vi "Dark Current Test Remastered Test Run.vi"() -> ()   [LabVIEW 2020]
uses:
  <instrlib>/CAEN PSM/CAEN PSM.lvlib
  <vilib>/Utility/file.llb/Write Delimited Spreadsheet (string).vi
  <vilib>/Utility/file.llb/Write Delimited Spreadsheet (DBL).vi
panel:
  out "7 4":bool
  out "6 4":bool
  out "8 4":bool
  out "5 4":bool
  out "4 4":bool
  out "3 4":bool
  out "2 4":bool
  out "1 4":bool
  out "Test is Running 4":bool
  out "OVV? 8":bool=TRUE
  out "OVC? 8":bool=TRUE
  out "Actual Voltage Level (V) 8":dbl format="%#_13g"
  out "Actual Current Limit (nA) 4":dbl format="%#_13g"
  in  "dt (s) 4":i32
  out "Time Left (s) 4":dbl
  out "Power Supply Trip 4":bool
  in  "N 4":i32
  in  "Channel # 4":i32
  in  "VISA resource name 4":refnum<visa-resource-name>
  out "OVV? 7":bool=TRUE
  out "OVC? 7":bool=TRUE
  out "Actual Voltage Level (V) 7":dbl format="%#_13g"
  out "Recorded Current\nfor Previous Tube 4":dbl format="%#_13g"
  in  "Measure Next Tube 4":bool
  out "Next Measurment 4":string
  in  "Barcodes 4":string[](array[string])
  out "Manual Measurments \nNeeded 4":bool
  in  "Begin Test 4":bool
  out "7 3":bool
  out "6 3":bool
  out "8 3":bool
  out "5 3":bool
  out "4 3":bool
  out "3 3":bool
  out "2 3":bool
  out "1 3":bool
  out "Test is Running 3":bool
  out "OVV? 6":bool=TRUE
  out "OVC? 6":bool=TRUE
  out "Actual Voltage Level (V) 6":dbl format="%#_13g"
  out "Actual Current Limit (nA) 3":dbl format="%#_13g"
  in  "dt (s) 3":i32
  out "Time Left (s) 3":dbl
  out "Power Supply Trip 3":bool
  in  "N 3":i32
  in  "Channel # 3":i32
  in  "VISA resource name 3":refnum<visa-resource-name>
  out "OVV? 5":bool=TRUE
  out "OVC? 5":bool=TRUE
  out "Actual Voltage Level (V) 5":dbl format="%#_13g"
  out "Recorded Current\nfor Previous Tube 3":dbl format="%#_13g"
  in  "Measure Next Tube 3":bool
  out "Next Measurment 3":string
  in  "Barcodes 3":string[](array[string])
  out "Manual Measurments \nNeeded 3":bool
  in  "Begin Test 3":bool
  out "7 2":bool
  out "6 2":bool
  out "8 2":bool
  out "5 2":bool
  out "4 2":bool
  out "3 2":bool
  out "2 2":bool
  out "1 2":bool
  out "Test is Running 2":bool
  out "OVV? 4":bool=TRUE
  out "OVC? 4":bool=TRUE
  out "Actual Voltage Level (V) 4":dbl format="%#_13g"
  out "Actual Current Limit (nA) 2":dbl format="%#_13g"
  in  "dt (s) 2":i32
  out "Time Left (s) 2":dbl
  out "Power Supply Trip 2":bool
  in  "N 2":i32
  in  "Channel # 2":i32
  in  "VISA resource name 2":refnum<visa-resource-name>
  out "OVV? 3":bool=TRUE
  out "OVC? 3":bool=TRUE
  out "Actual Voltage Level (V) 3":dbl format="%#_13g"
  out "Recorded Current\nfor Previous Tube 2":dbl format="%#_13g"
  in  "Measure Next Tube 2":bool
  out "Next Measurment 2":string
  in  "Barcodes 2":string[](array[string])
  out "Manual Measurments \nNeeded 2":bool
  in  "Begin Test 2":bool
  out "Power Supply Trip":bool
  out "Time Left (s)":dbl
  out "8":bool
  out "7":bool
  out "6":bool
  out "5":bool
  out "4":bool
  out "3":bool
  out "2":bool
  out "1":bool
  out "Test is Running":bool
  in  "Begin Test":bool
  out "Manual Measurments \nNeeded":bool
  out "OVV? 2":bool=TRUE
  out "OVC? 2":bool=TRUE
  out "Actual Voltage Level (V) 2":dbl format="%#_13g"
  out "Recorded Current\nfor Previous Tube":dbl format="%#_13g"
  in  "Measure Next Tube":bool
  in  "Barcodes":string[](array[string])
  out "Next Measurment":string
  in  "N":i32
  in  "dt (s)":i32
  out "Actual Current Limit (nA)":dbl format="%#_13g"
  out "Actual Voltage Level (V)":dbl format="%#_13g"
  out "OVC?":bool=TRUE
  out "OVV?":bool=TRUE
  in  "Channel #":i32
  in  "VISA resource name":refnum<visa-resource-name>
  # "Dark Current Test"
  # "Instructions in Brief:\n1. Begin the program by clicking the white arrow.\n2. Assemble tubes into the test bench.\n3. Select COM5 for the \"VISA resource name\".\n4. Enter in how often you want to take measurement in the \"dt\" box (typically 60s)\n5. Enter in how many measurments you want to take (typically 15)\n6. Scan in the 8 tubes that you are testing.\n(If you take 15 measurments every 60s, the test will take 15 min.)\n7. Click \"Begin Test\". The \"Test is Running\" LED should light up.\n8. After the intial test, if the total current is below 16nA, \n    the program will write the \n     file and end the test.\n9. If the total current is above 16nA, manual\n    measurments need to be taken.\n10. Engage only the tube indicated by \"Next Measurment\". \n11. Click \"Measure\".\n12. Engage the next tube and continue untill all have been measured.\n13. In both cases, the program will write files and end the test. \n14. The test is over when the \"Test is Running\" LED has turned off."
  # "Green lights indicate tubes that have passed."
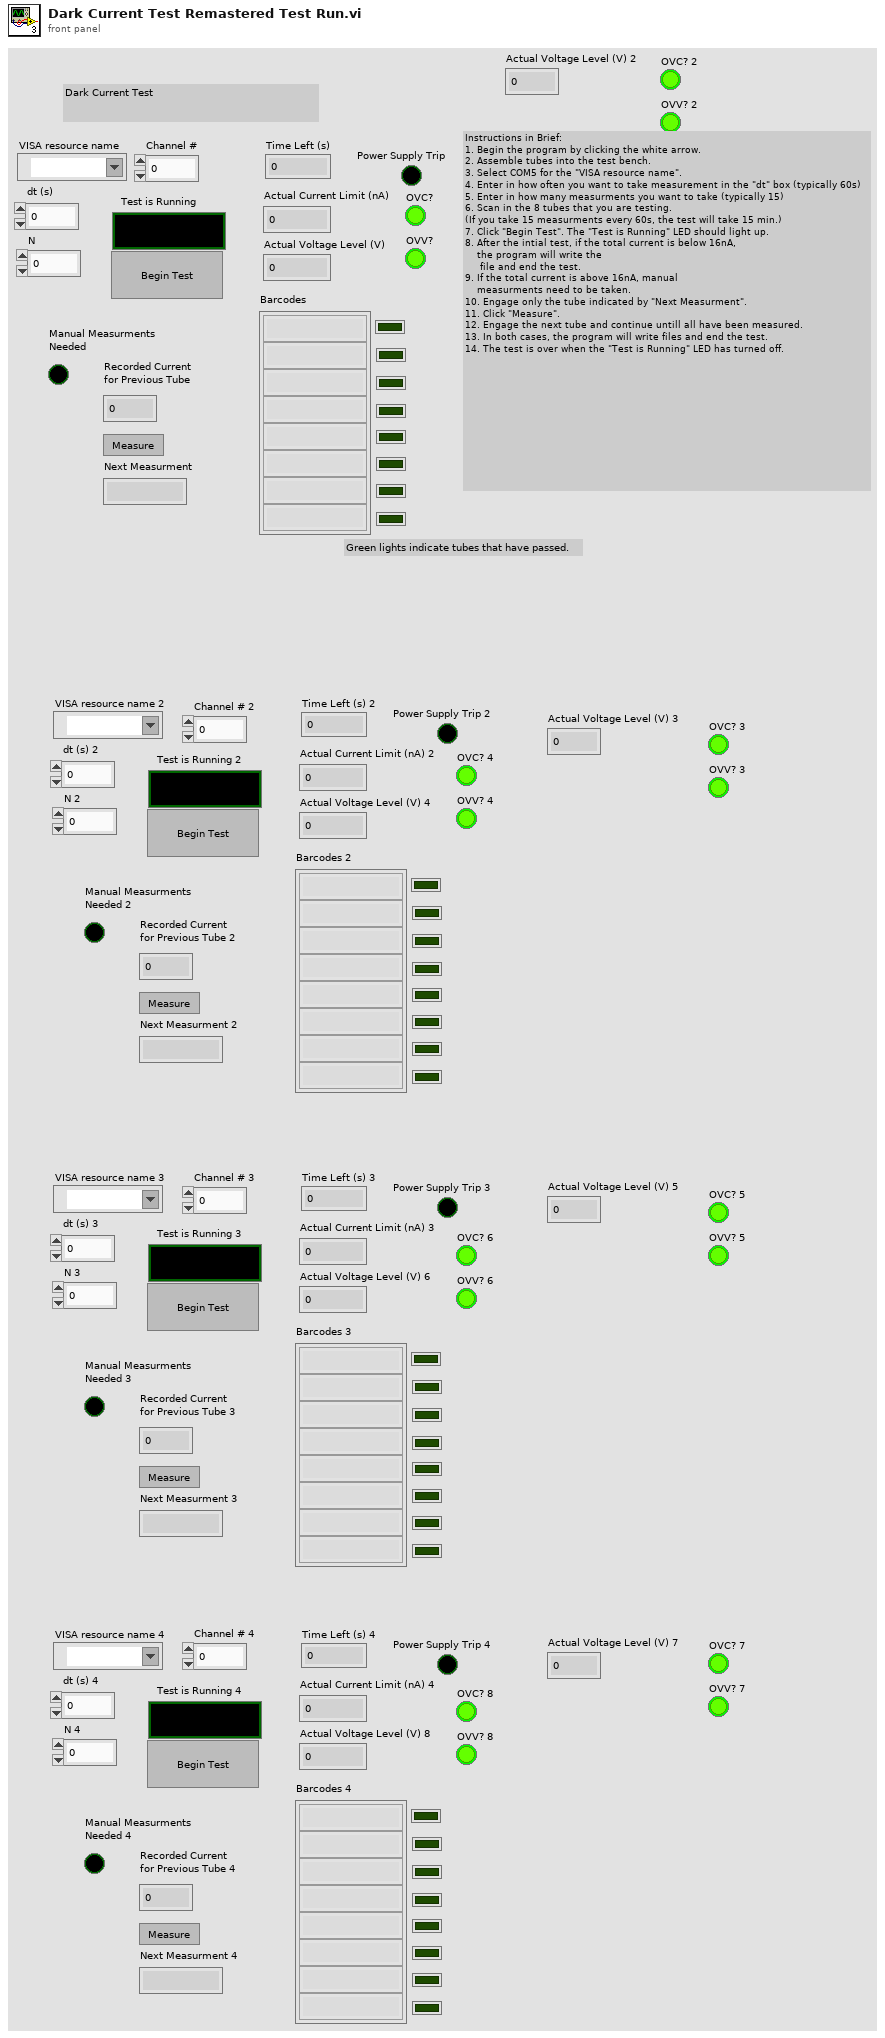
[diagram p1: front panel]
types:
  T1 = cluster{"VISA resource name":refnum<visa-resource-name>, "Board address":u8, "NChannels":u8}
  T2 = cluster{"ON":bool, "RUP":bool, "RDW":bool, "OVC":bool, "OVV":bool, "UNV":bool, "MAXV":bool, "TRIP":bool, "OVP":bool, "OVT":bool, "DIS":bool, "KILL":bool, "ILK":bool, "NOCAL":bool}[]
  T3 = cluster{"ON":bool, "RUP":bool, "RDW":bool, "OVC":bool, "OVV":bool, "UNV":bool, "MAXV":bool, "TRIP":bool, "OVP":bool, "OVT":bool, "DIS":bool, "KILL":bool, "ILK":bool, "NOCAL":bool}
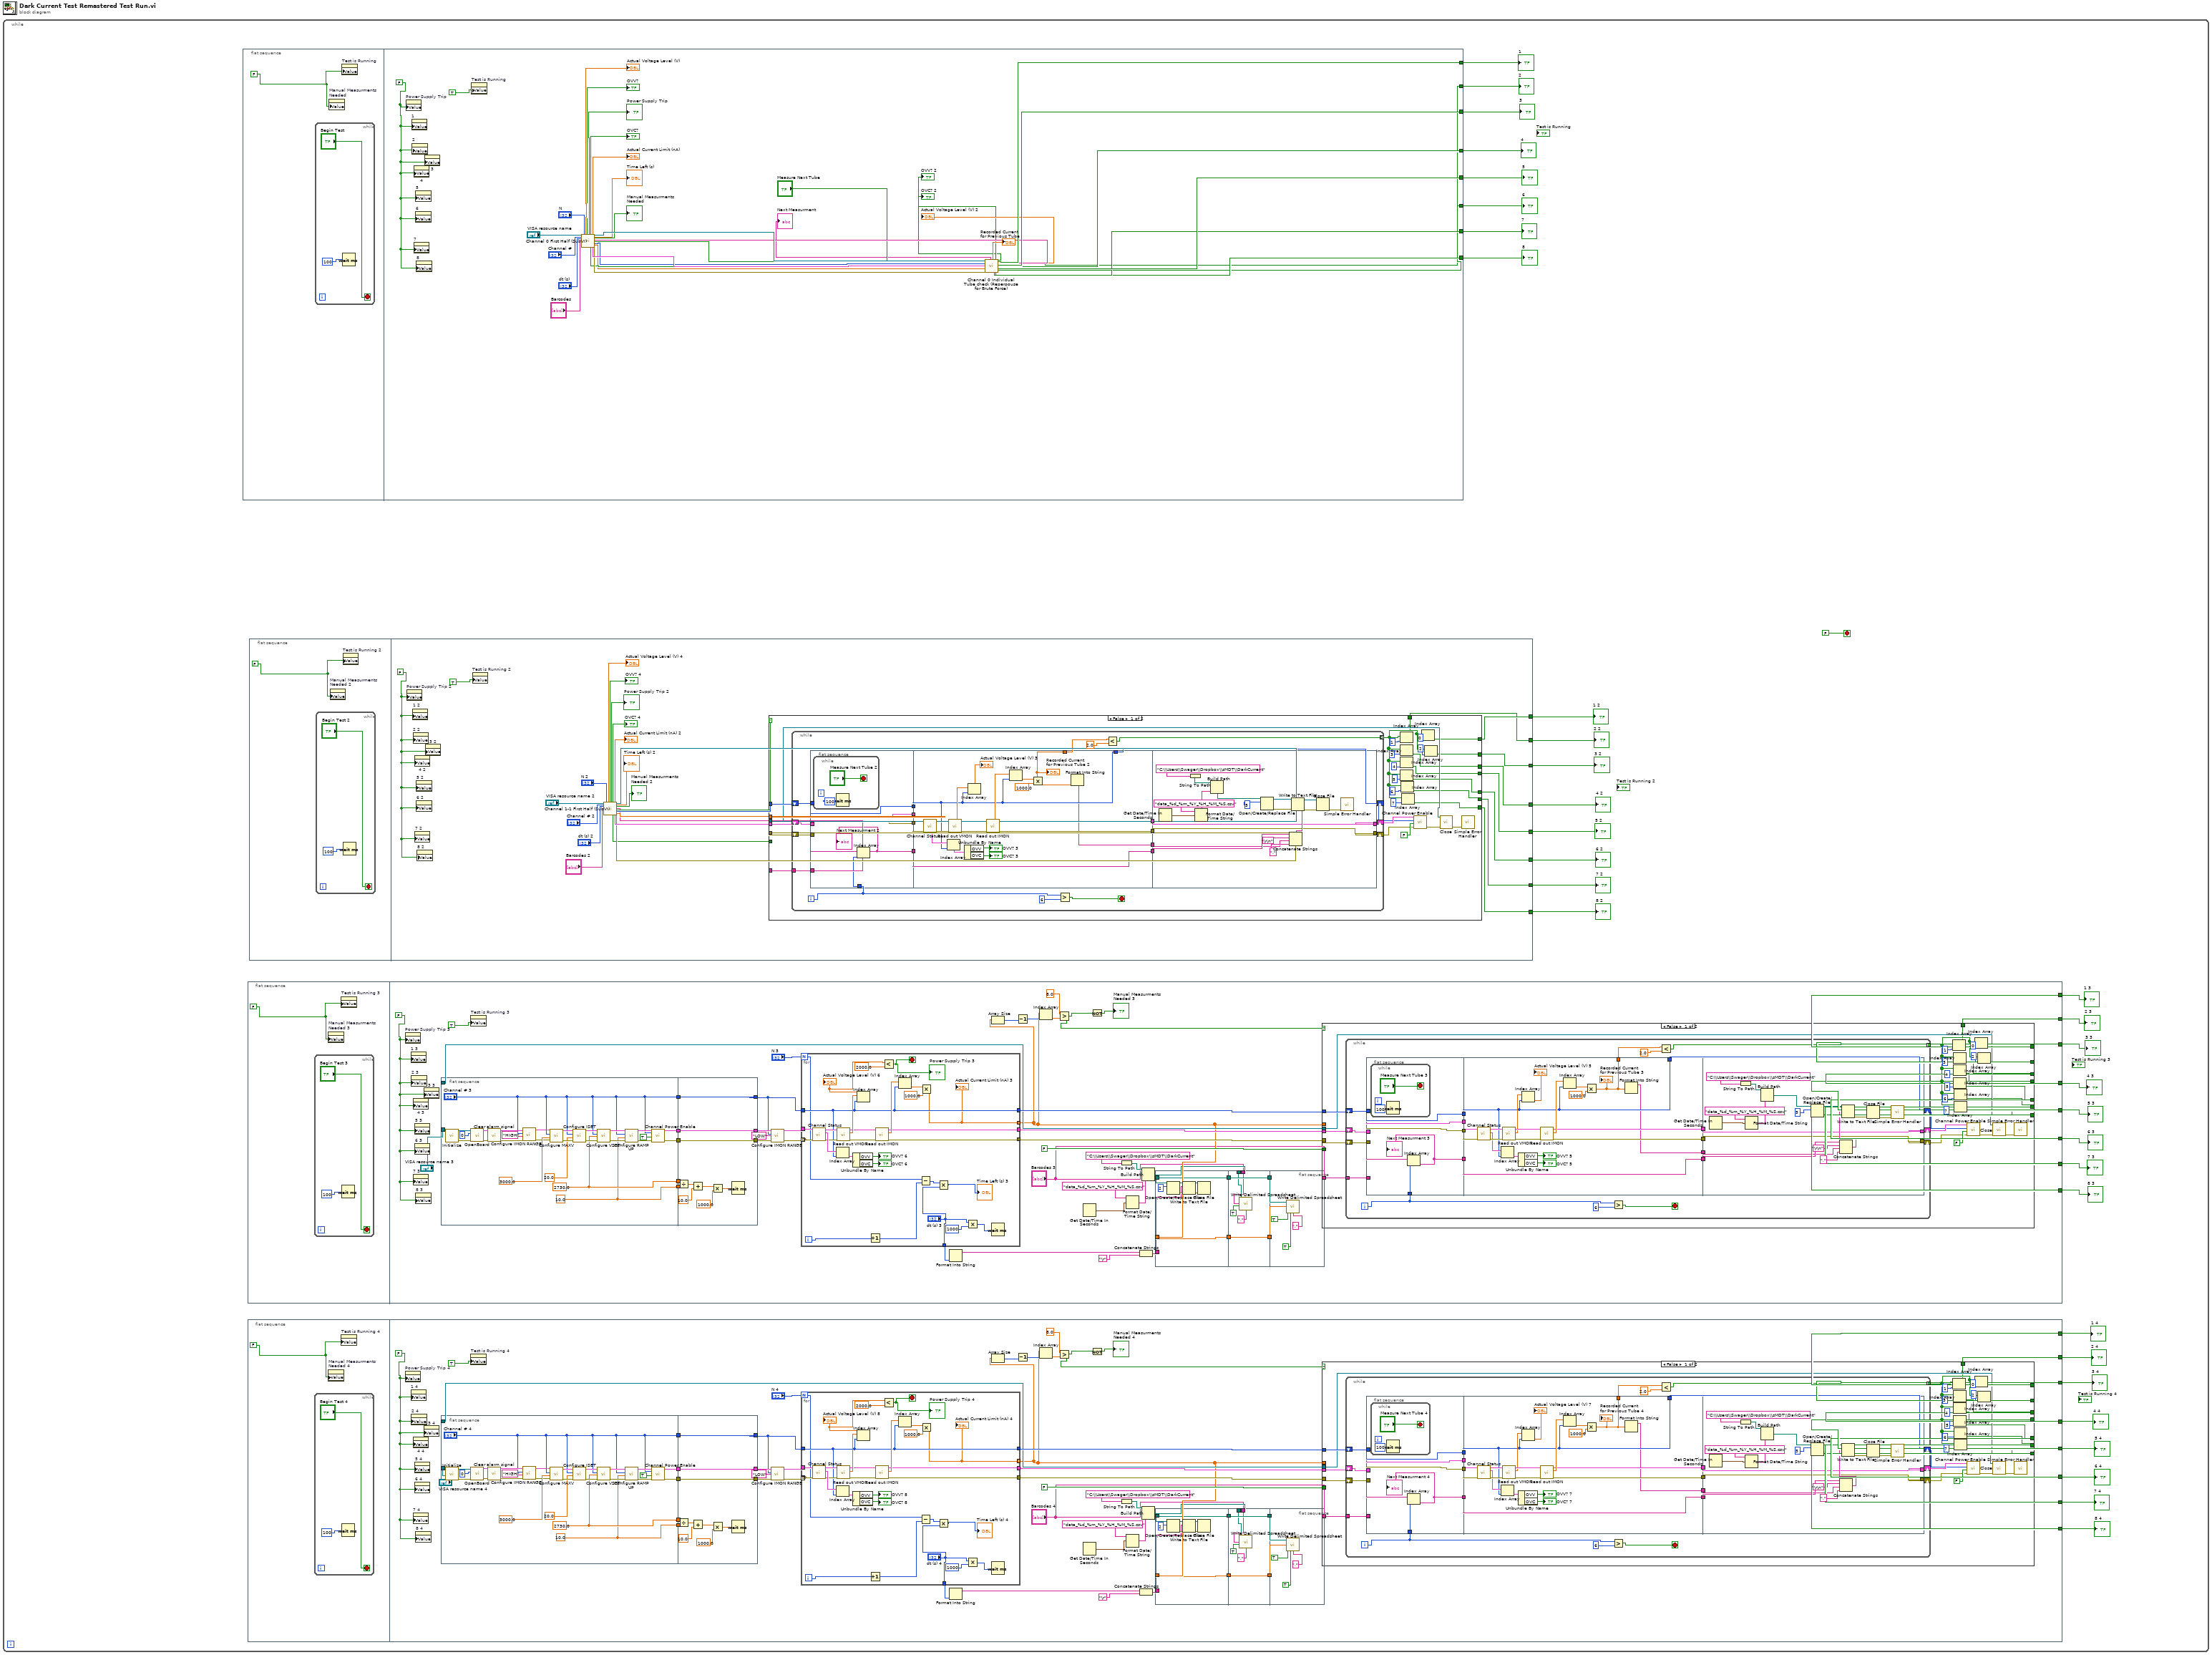
[diagram p0: block diagram]
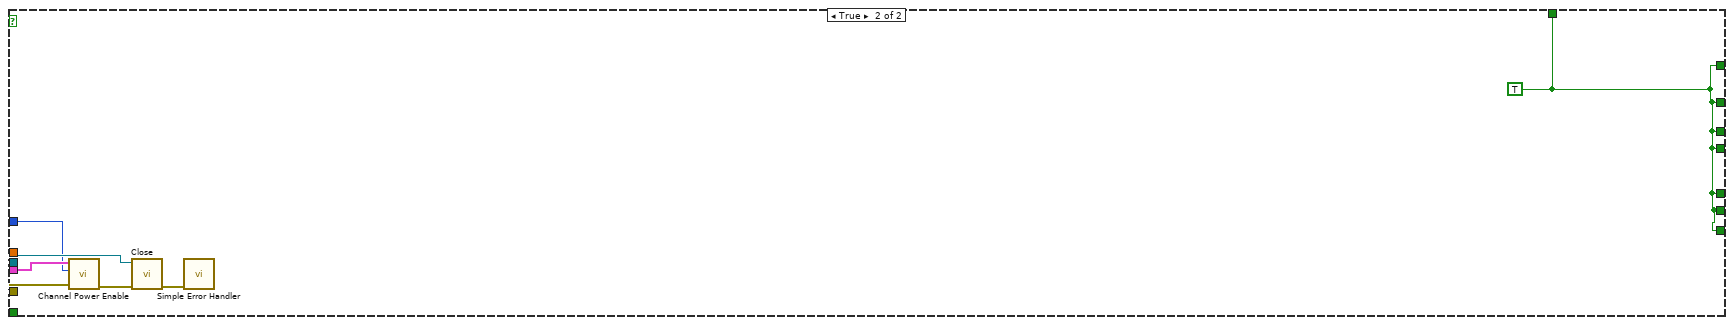
[diagram p2: hidden frame]
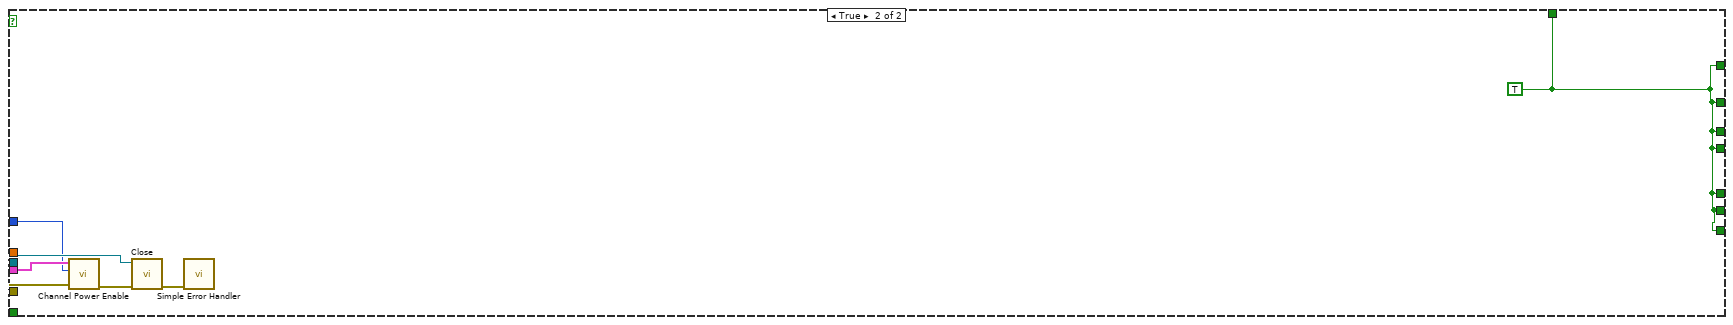
[diagram p3: hidden frame]
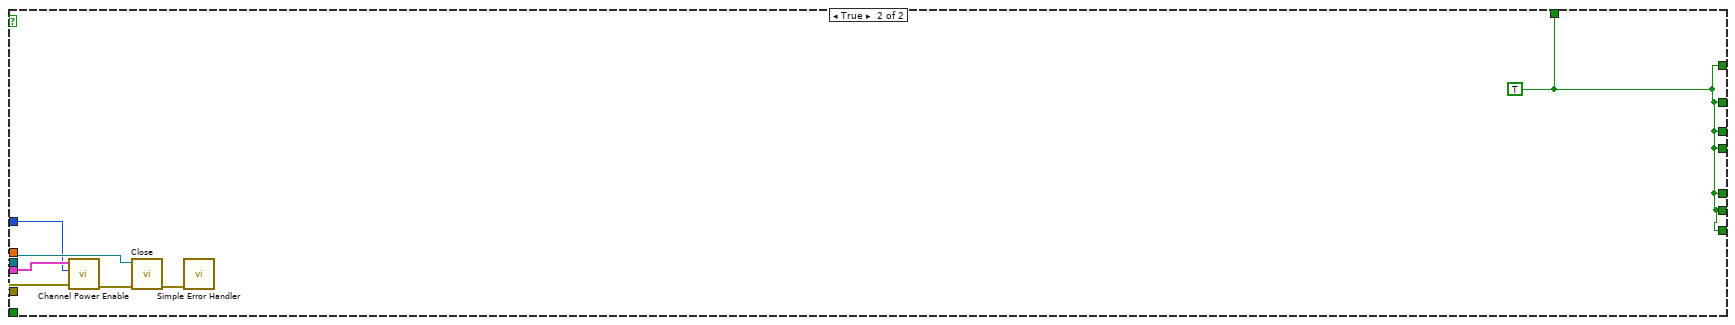
[diagram p4: hidden frame]
diagram:
  n1 = while {
    stop <- FALSE stop-if-true
    n2 = flat-sequence {
      tunnel: [w684] -> w32
      tunnel: [w664] -> w31
      tunnel: [w683] -> w30
      tunnel: [w682] -> w29
      tunnel: [w681] -> w28
      tunnel: [w665] -> w27
      tunnel: [w680] -> w26
      tunnel: [w679] -> w25
      frame #0 {
        w655 = FALSE
        n3 = while {
          stop <- "Begin Test" stop-if-true
          n4 = Wait (ms)(milliseconds to wait=100) -> ()  [unwired: 1 out]
        }
        n5 = property on="Manual Measurments \nNeeded" class="Bool (strict)"("Value"=w655) -> ()  [unwired: 2 in, 2 out]
        n6 = property on="Test is Running" class="Bool (strict)"("Value"=w655) -> ()  [unwired: 2 in, 2 out]
      }
      frame #1 {
        w677 = FALSE
        n7 = property on="Power Supply Trip" class="Bool (strict)"("Value"=w677) -> ()  [unwired: 2 in, 2 out]
        n8 = property on="1" class="Bool (strict)"("Value"=w677) -> ()  [unwired: 2 in, 2 out]
        n9 = property on="2" class="Bool (strict)"("Value"=w677) -> ()  [unwired: 2 in, 2 out]
        n10 = property on="4" class="Bool (strict)"("Value"=w677) -> ()  [unwired: 2 in, 2 out]
        n11 = property on="7" class="Bool (strict)"("Value"=w677) -> ()  [unwired: 2 in, 2 out]
        n12 = property on="5" class="Bool (strict)"("Value"=w677) -> ()  [unwired: 2 in, 2 out]
        n13 = property on="6" class="Bool (strict)"("Value"=w677) -> ()  [unwired: 2 in, 2 out]
        n14 = property on="8" class="Bool (strict)"("Value"=w677) -> ()  [unwired: 2 in, 2 out]
        n15 = property on="3" class="Bool (strict)"("Value"=w677) -> ()  [unwired: 2 in, 2 out]
        n16 = property on="Test is Running" class="Bool (strict)"("Value"=TRUE) -> ()  [unwired: 2 in, 2 out]
        n17 = call "Channel 0 First Half (SubVI).vi"("VISA Refnum in"="VISA resource name", "Channel #"="Channel #", "dt (s)"="dt (s)", "Barcodes in"="Barcodes", "N"="N") -> ("Actual Voltage Level (V)"=→"Actual Voltage Level (V)":dbl, "OVV?"=→"OVV?":bool, "Power Supply Trip"=→"Power Supply Trip":bool, "OVC?"=→"OVC?":bool, "Boolean 2"=w690:bool, "Actual Current Limit (nA)"=→"Actual Current Limit (nA)":dbl, "BoardHandle out 2"=w692:T1, "VISA Refnum out"=w688:refnum<visa-resource-name>, "Time Left (s)"=→"Time Left (s)":dbl, "Manual Measurments \nNeeded"=→"Manual Measurments \nNeeded":bool, "Barcodes out"=w676:string[], "Boolean"=w686:bool, "Channel # out 2"=w689:i32, "Array"=w678:dbl[], "error out"=w691:errorcluster)  [unwired: 8 in]
        n18 = call "Channel 0 Individual Tube check (Reperpouse for Brute Force).vi"("VISA Refnum in"=w688, "Boolean 9"=w686, "Channel # in"=w689, "BoardHandle in"=w692, "Boolean 10"=w690, "Array"=w678, "error in (no error)"=w691, "Barcodes in"=w676, 10:"Measure Next Tube") -> ("Next Measurment"=→"Next Measurment":string, "Recorded Current\nfor Previous Tube"=→"Recorded Current\nfor Previous Tube":dbl, "Actual Voltage Level (V) 2"=→"Actual Voltage Level (V) 2":dbl, "Boolean 3"=w679:bool, "OVC? 2"=→"OVC? 2":bool, "Boolean 4"=w680:bool, "OVV? 2"=→"OVV? 2":bool, "Boolean 8"=w684:bool, "Boolean"=w664:bool, "Boolean 7"=w683:bool, "Boolean 6"=w682:bool, "Boolean 5"=w681:bool, "Boolean 2"=w665:bool)  [unwired: 6 in]
      }
    }
    n19 = flat-sequence {
      tunnel: [w303] -> w16
      tunnel: [w302] -> w15
      tunnel: [w301] -> w14
      tunnel: [w300] -> w13
      tunnel: [w299] -> w12
      tunnel: [w298] -> w11
      tunnel: [w297] -> w10
      tunnel: [w296] -> w9
      frame #0 {
        w276 = FALSE
        n20 = while {
          stop <- "Begin Test 3" stop-if-true
          n21 = Wait (ms)(milliseconds to wait=100) -> ()  [unwired: 1 out]
        }
        n22 = property on="Manual Measurments \nNeeded 3" class="Bool (strict)"("Value"=w276) -> ()  [unwired: 2 in, 2 out]
        n23 = property on="Test is Running 3" class="Bool (strict)"("Value"=w276) -> ()  [unwired: 2 in, 2 out]
      }
      frame #1 {
        w289 = FALSE
        n24 = property on="Power Supply Trip 3" class="Bool (strict)"("Value"=w289) -> ()  [unwired: 2 in, 2 out]
        n25 = property on="1 3" class="Bool (strict)"("Value"=w289) -> ()  [unwired: 2 in, 2 out]
        n26 = property on="2 3" class="Bool (strict)"("Value"=w289) -> ()  [unwired: 2 in, 2 out]
        n27 = property on="4 3" class="Bool (strict)"("Value"=w289) -> ()  [unwired: 2 in, 2 out]
        n28 = property on="7 3" class="Bool (strict)"("Value"=w289) -> ()  [unwired: 2 in, 2 out]
        n29 = property on="5 3" class="Bool (strict)"("Value"=w289) -> ()  [unwired: 2 in, 2 out]
        n30 = property on="6 3" class="Bool (strict)"("Value"=w289) -> ()  [unwired: 2 in, 2 out]
        n31 = property on="8 3" class="Bool (strict)"("Value"=w289) -> ()  [unwired: 2 in, 2 out]
        n32 = property on="3 3" class="Bool (strict)"("Value"=w289) -> ()  [unwired: 2 in, 2 out]
        n33 = flat-sequence {
          tunnel: [w463] -> w328
          tunnel: [w462] -> w327
          tunnel: [w459] -> w318
          tunnel: [w461] -> w326
          tunnel: [w460] -> w325
          tunnel: ["Channel # 3"] -> w324
          tunnel: "VISA resource name 3" -> [w459]
          tunnel: w328 -> [w483]
          tunnel: w327 -> [w482]
          tunnel: [w481] -> w315
          tunnel: w326 -> [w481]
          tunnel: [w480] -> w316
          tunnel: w325 -> [w480]
          tunnel: [w479] -> w313
          tunnel: w324 -> [w479]
          frame #0 {
            w463 = 2730.0 ("Voltage Set (Volts)")
            w462 = 10.0 ("Voltage Ramp Up (V/s)")
            n34 = call <instrlib>:"Initialize.vi"("VISA resource name"=w459) -> ("error out"=w473:errorcluster, "VISA resource name out"=w469:refnum<visa-resource-name>)  [unwired: 9 in]
            n35 = call <instrlib>:"OpenBoard.vi"("error in (no error)"=w473, "Board Address"=0, "VISA resource name"=w469) -> ("error out"=w474:errorcluster, "BoardHandle"=w468:T1)  [unwired: 7 in]
            n36 = call <instrlib>:"Clear alarm signal.vi"("error in (no error)"=w474, "BoardHandle"=w468) -> ("error out"=w457:errorcluster, "BoardHandle out"=w456:T1)  [unwired: 8 in]
            n37 = call <instrlib>:"Configure IMON RANGE.vi"("error in (no error)"=w457, "IMon range (LOW)"="HIGH", "Channel (0)"="Channel # 3", "BoardHandle"=w456) -> ("error out"=w452:errorcluster, "BoardHandle out"=w453:T1)  [unwired: 6 in]
            n38 = call <instrlib>:"Configure MAXV.vi"("error in (no error)"=w452, "Voltage Max (0.0 V)"=3000.0 ("VMax (Volts)"), "Channel (0)"="Channel # 3", "BoardHandle"=w453) -> ("error out"=w475:errorcluster, "BoardHandle out"=w467:T1)  [unwired: 6 in]
            n39 = call <instrlib>:"Configure ISET.vi"("error in (no error)"=w475, "Current Limit (0.00 uA)"=20.0 ("Current Limit (uA)"), "Channel (0)"="Channel # 3", "BoardHandle"=w467) -> ("error out"=w476:errorcluster, "BoardHandle out"=w466:T1)  [unwired: 6 in]
            n40 = call <instrlib>:"Configure VSET.vi"("error in (no error)"=w476, "Voltage Level (0.0 V)"=w463, "Channel (0)"="Channel # 3", "BoardHandle"=w466) -> ("error out"=w477:errorcluster, "BoardHandle out"=w465:T1)  [unwired: 6 in]
            n41 = call <instrlib>:"Configure RAMP UP.vi"("error in (no error)"=w477, "Voltage ramp up (0 V/s)"=w462, "Channel (0)"="Channel # 3", "BoardHandle"=w465) -> ("error out"=w478:errorcluster, "BoardHandle out"=w464:T1)  [unwired: 6 in]
            n42 = call <instrlib>:"Channel Power Enable.vi"("error in (no error)"=w478, "Enable (OFF)"=TRUE ("Boolean"), "Channel (0)"="Channel # 3", "BoardHandle"=w464) -> ("error out"=w460:errorcluster, "BoardHandle out"=w461:T1)  [unwired: 6 in]
          }
          frame #1 {
            n43 = Divide(x=w483, y=w482) -> (x/y=w486:dbl)
            n44 = Add(x=w486, y=10.0) -> (x+y=w487:dbl)
            n45 = Multiply(x=w487, y=1000.0) -> (x*y=w488:dbl)
            n46 = Wait (ms)(milliseconds to wait=w488) -> ()  [unwired: 1 out]
          }
        }
        n47 = property on="Test is Running 3" class="Bool (strict)"("Value"=TRUE) -> ()  [unwired: 2 in, 2 out]
        n48 = call <instrlib>:"Configure IMON RANGE.vi"("error in (no error)"=w316, "IMon range (LOW)"="LOW", "Channel (0)"=w313, "BoardHandle"=w315) -> ("error out"=w311:errorcluster, "BoardHandle out"=w312:T1)  [unwired: 6 in]
        n49 = for {
          N: "N 3" -> [w497]
          tunnel: w311 -> [w504]
          tunnel: w313 -> [w505]
          tunnel: [w507] -> w322
          tunnel: [w506] -> w321
          tunnel: [w498] -> w290 mode=indexing
          tunnel: [w505] -> w319
          tunnel: w312 -> [w501]
          tunnel: [w504] -> _ mode=indexing
          tunnel: ["dt (s) 3"] -> w288
          i -> [w494]
          stop <- w492 stop-if-true
          n50 = call <instrlib>:"Channel Status.vi"("error in (no error)"=w504, "BoardHandle"=w501) -> ("error out"=w513:errorcluster, "Channel Status Array"=w517:T2, "BoardHandle out"=w512:T1)  [unwired: 7 in]
          n51 = Index Array(array=w517, index=w505) -> (element=w516:T3)
          n52 = call <instrlib>:"Read out VMON.vi"("error in (no error)"=w513, "BoardHandle"=w512) -> ("error out"=w509:errorcluster, "VMon values (V)"=w511:dbl[], "BoardHandle out"=w510:T1)  [unwired: 7 in]
          n53 = Unbundle By Name(w516) -> ("OVV"=→"OVV? 6":bool, "OVC"=→"OVC? 6":bool)
          n54 = Index Array(array=w511, index=w505) -> (element=w491:dbl)
          "Actual Voltage Level (V) 6" <- w491
          n55 = Increment(x=w494) -> (x+1=w493:i32)
          n56 = call <instrlib>:"Read out IMON.vi"("error in (no error)"=w509, "BoardHandle"=w510) -> ("error out"=w506:errorcluster, "IMon values (uA)"=w508:dbl[], "BoardHandle out"=w507:T1)  [unwired: 6 in, 1 out]
          n57 = Less?(x=w491, y=2000.0) -> (x < y?=w492:bool)
          "Power Supply Trip 3" <- w492
          n58 = Index Array(array=w508, index=w505) -> (element=w500:dbl)
          n59 = Subtract(x=w497, y=w493) -> (x-y=w496:i32)
          n60 = Multiply(x=w500, y=1000.0) -> (x*y=w498:dbl)
          "Actual Current Limit (nA) 3" <- w498
          n61 = Multiply(x=w496, y="dt (s) 3") -> (x*y=→"Time Left (s) 3":i32)
          n62 = Multiply(x="dt (s) 3", y=1000) -> (x*y=w503:i32)
          n63 = Wait (ms)(milliseconds to wait=w503) -> ()  [unwired: 1 out]
        }
        n64 = Format Into String(w288) -> (resulting string=w280:string)  [unwired: 3 in, 1 out]
        n65 = Array Size(array=w290) -> (size(s)=w310:i32)
        n66 = Decrement(x=w310) -> (x-1=w309:i32)
        n67 = Index Array(array=w290, index=w309) -> (element=w308:dbl)
        n68 = Greater?(x=8.0, y=w308) -> (0:w307:bool)
        n69 = Get Date/Time In Seconds() -> (seconds since 1Jan1904=w293:timestamp)
        n70 = Not(x=w307) -> (.not. x?=→"Manual Measurments \nNeeded 3":bool)
        n71 = String To Path(string="C:\\Users\\Swager\\Dropbox\\sMDT\\DarkCurrent") -> (path=w292:path)
        n72 = Format Date/Time String(time format string (%c)="data_%d_%m_%Y_%H_%M_%S.csv", seconds (now)=w293) -> (date/time string=w294:string)  [unwired: 1 in]
        n73 = Concatenate Strings(w280, "\r") -> (w281:string)
        n74 = Build Path(base path=w292, name or relative path=w294) -> (appended path=w283:path)
        n75 = flat-sequence {
          tunnel: w283 -> [w335]
          tunnel: [w335] -> w287
          tunnel: [w336] -> w285
          tunnel: w290 -> [w336]
          tunnel: w281 -> [w332]
          tunnel: w287 -> [w342]
          tunnel: [w342] -> w286
          tunnel: w285 -> [w341]
          tunnel: [w341] -> w284
          tunnel: w283 -> [w340]
          tunnel: "Barcodes 3" -> [w339]
          tunnel: w286 -> [w345]
          tunnel: w284 -> [w344]
          frame #0 {
            n76 = Open/Create/Replace File(file path (use dialog)=w335, operation (0:open)=2) -> (refnum out=w333:refnum<file>, error out=w334:errorcluster)  [unwired: 4 in, 1 out]
            n77 = Write to Text File(file (use dialog)=w333, text=w332, error in=w334) -> (refnum out=w330:refnum<file>, error out=w331:errorcluster)  [unwired: 1 in, 1 out]
            n78 = Close File(refnum=w330, error in=w331) -> ()  [unwired: 2 out]
          }
          frame #1 {
            n79 = call-poly <vilib>:"Write Delimited Spreadsheet.vi"("file path (dialog if empty)"=w340, "1D data"=w339, "append to file? (new file:F)"=TRUE, "delimiter (\\t)"=",") -> ()  [unwired: 10 in, 2 out]
          }
          frame #2 {
            n80 = call-poly <vilib>:"Write Delimited Spreadsheet.vi"("file path (dialog if empty)"=w345, "1D data"=w344, "append to file? (new file:F)"=TRUE, "transpose? (no:F)"=TRUE, "delimiter (\\t)"=",") -> ()  [unwired: 9 in, 2 out]
          }
        }
        n81 = case shown="False" w307 {
          tunnel: w322 -> [w374 w447]
          tunnel: w321 -> [w375 w446]
          tunnel: FALSE -> [_ _]
          tunnel: w319 -> [w373 w445]
          tunnel: w318 -> [w369 w448]
          tunnel: w290 -> [_ _]
          tunnel: "Barcodes 3" -> [w365 _]
          tunnel: [w355 w451] -> w303
          tunnel: [w354 w451] -> w302
          tunnel: [w353 w451] -> w301
          tunnel: [w352 w451] -> w300
          tunnel: [w351 w451] -> w299
          tunnel: [w350 w451] -> w298
          tunnel: [w349 w451] -> w297
          tunnel: [w348 w451] -> w296
          frame False {
            n82 = while {
              shift-right: [w381] -> w366
              shift-left: w373 -> [w391]
              shift-right: [w383] -> w368
              shift-left: w374 -> [w388]
              shift-right: [w382] -> w367
              shift-left: w375 -> [w386]
              tunnel: w365 -> [w379]
              tunnel: [w376] -> w364 mode=indexing
              i -> [w394]
              stop <- w395 stop-if-true
              n83 = flat-sequence {
                tunnel: w394 -> [w402]
                tunnel: [w401] -> w393
                tunnel: w391 -> [w400]
                tunnel: [w400] -> w390
                tunnel: [w399] -> w389
                tunnel: w388 -> [w399]
                tunnel: [w398] -> w387
                tunnel: w386 -> [w398]
                tunnel: w379 -> [w397]
                tunnel: w393 -> [w412]
                tunnel: [w412] -> w392
                tunnel: w390 -> [w407]
                tunnel: w389 -> [w410]
                tunnel: w387 -> [w411]
                tunnel: [w409] -> w385
                tunnel: [w408] -> w384
                tunnel: [w407] -> w381
                tunnel: [w406] -> w380
                tunnel: [w405] -> w378
                tunnel: w392 -> [w430]
                tunnel: w385 -> [w428]
                tunnel: w384 -> [w427]
                tunnel: [w428] -> w383
                tunnel: [w427] -> w382
                tunnel: w380 -> [w426]
                frame #0 {
                  n84 = while {
                    stop <- "Measure Next Tube 3" stop-if-true
                    n85 = Wait (ms)(milliseconds to wait=100) -> ()  [unwired: 1 out]
                  }
                  n86 = Index Array(array=w397, index=w402) -> (element=w401:string)
                  "Next Measurment 3" <- w401
                }
                frame #1 {
                  n87 = call <instrlib>:"Channel Status.vi"("error in (no error)"=w411, "BoardHandle"=w410) -> ("error out"=w418:errorcluster, "Channel Status Array"=w414:T2, "BoardHandle out"=w419:T1)  [unwired: 7 in]
                  n88 = Index Array(array=w414, index=w407) -> (element=w415:T3)
                  n89 = call <instrlib>:"Read out VMON.vi"("error in (no error)"=w418, "BoardHandle"=w419) -> ("error out"=w422:errorcluster, "VMon values (V)"=w420:dbl[], "BoardHandle out"=w421:T1)  [unwired: 7 in]
                  n90 = Unbundle By Name(w415) -> ("OVV"=→"OVV? 5":bool, "OVC"=→"OVC? 5":bool)
                  n91 = Index Array(array=w420, index=w407) -> (element=→"Actual Voltage Level (V) 5":dbl)
                  n92 = call <instrlib>:"Read out IMON.vi"("error in (no error)"=w422, "BoardHandle"=w421) -> ("error out"=w408:errorcluster, "IMon values (uA)"=w425:dbl[], "BoardHandle out"=w409:T1)  [unwired: 6 in, 1 out]
                  n93 = Index Array(array=w425, index=w407) -> (element=w423:dbl)
                  n94 = Multiply(x=w423, y=1000.0) -> (x*y=w405:dbl)
                  "Recorded Current\nfor Previous Tube 3" <- w405
                  n95 = Format Into String(w405) -> (resulting string=w406:string)  [unwired: 3 in, 1 out]
                }
                frame #2 {
                  n96 = Get Date/Time In Seconds() -> (seconds since 1Jan1904=w442:timestamp)
                  n97 = String To Path(string="C:\\Users\\Swager\\Dropbox\\sMDT\\DarkCurrent") -> (path=w441:path)
                  n98 = Format Date/Time String(time format string (%c)="data_%d_%m_%Y_%H_%M_%S.csv", seconds (now)=w442) -> (date/time string=w443:string)  [unwired: 1 in]
                  n99 = Build Path(base path=w441, name or relative path=w443) -> (appended path=w439:path)
                  n100 = Open/Create/Replace File(file path (use dialog)=w439, operation (0:open)=5) -> (refnum out=w438:refnum<file>, error out=w437:errorcluster)  [unwired: 4 in, 1 out]
                  n101 = Concatenate Strings(w430, "\r\n", w426, ",") -> (w432:string)
                  n102 = Write to Text File(file (use dialog)=w438, text=w432, error in=w437) -> (refnum out=w436:refnum<file>, error out=w435:errorcluster)  [unwired: 1 in, 1 out]
                  n103 = Close File(refnum=w436, error in=w435) -> (error out=w434:errorcluster)  [unwired: 1 out]
                  n104 = call <vilib>:"Simple Error Handler.vi"("error in (no error)"=w434) -> ()  [unwired: 4 in, 5 out]
                }
              }
              n105 = Greater?(x=w394, y=6) -> (0:w395:bool)
              n106 = Less?(x=w378, y=2.0) -> (x < y?=w376:bool)
            }
            n107 = Index Array(array=w364, index=1) -> (element=w354:bool)
            n108 = Index Array(array=w364, index=3) -> (element=w352:bool)
            n109 = Index Array(array=w364, index=4) -> (element=w351:bool)
            n110 = Index Array(array=w364, index=5) -> (element=w350:bool)
            n111 = Index Array(array=w364, index=6) -> (element=w349:bool)
            n112 = Index Array(array=w364, index=7) -> (element=w348:bool)
            n113 = call <instrlib>:"Channel Power Enable.vi"("error in (no error)"=w367, "Enable (OFF)"=FALSE, "Channel (0)"=w366, "BoardHandle"=w368) -> ("error out"=w371:errorcluster)  [unwired: 6 in, 1 out]
            n114 = Index Array(array=w364, index=0) -> (element=w355:bool)
            n115 = Index Array(array=w364, index=2) -> (element=w353:bool)
            n116 = call <instrlib>:"Close.vi"("error in (no error)"=w371, "VISA resource name"=w369) -> ("error out"=w370:errorcluster)  [unwired: 9 in]
            n117 = call <vilib>:"Simple Error Handler.vi"("error in (no error)"=w370) -> ()  [unwired: 4 in, 5 out]
          }
          frame True {
            w451 = TRUE
            n118 = call <instrlib>:"Channel Power Enable.vi"("error in (no error)"=w446, "Channel (0)"=w445, "BoardHandle"=w447) -> ("error out"=w450:errorcluster)  [unwired: 7 in, 1 out]
            n119 = call <instrlib>:"Close.vi"("error in (no error)"=w450, "VISA resource name"=w448) -> ("error out"=w449:errorcluster)  [unwired: 9 in]
            n120 = call <vilib>:"Simple Error Handler.vi"("error in (no error)"=w449) -> ()  [unwired: 4 in, 5 out]
          }
        }
      }
    }
    n121 = flat-sequence {
      tunnel: [w61] -> w8
      tunnel: [w60] -> w7
      tunnel: [w59] -> w6
      tunnel: [w58] -> w5
      tunnel: [w57] -> w4
      tunnel: [w56] -> w3
      tunnel: [w55] -> w2
      tunnel: [w54] -> w1
      frame #0 {
        w34 = FALSE
        n122 = while {
          stop <- "Begin Test 4" stop-if-true
          n123 = Wait (ms)(milliseconds to wait=100) -> ()  [unwired: 1 out]
        }
        n124 = property on="Manual Measurments \nNeeded 4" class="Bool (strict)"("Value"=w34) -> ()  [unwired: 2 in, 2 out]
        n125 = property on="Test is Running 4" class="Bool (strict)"("Value"=w34) -> ()  [unwired: 2 in, 2 out]
      }
      frame #1 {
        w47 = FALSE
        n126 = property on="Power Supply Trip 4" class="Bool (strict)"("Value"=w47) -> ()  [unwired: 2 in, 2 out]
        n127 = property on="1 4" class="Bool (strict)"("Value"=w47) -> ()  [unwired: 2 in, 2 out]
        n128 = property on="2 4" class="Bool (strict)"("Value"=w47) -> ()  [unwired: 2 in, 2 out]
        n129 = property on="4 4" class="Bool (strict)"("Value"=w47) -> ()  [unwired: 2 in, 2 out]
        n130 = property on="7 4" class="Bool (strict)"("Value"=w47) -> ()  [unwired: 2 in, 2 out]
        n131 = property on="5 4" class="Bool (strict)"("Value"=w47) -> ()  [unwired: 2 in, 2 out]
        n132 = property on="6 4" class="Bool (strict)"("Value"=w47) -> ()  [unwired: 2 in, 2 out]
        n133 = property on="8 4" class="Bool (strict)"("Value"=w47) -> ()  [unwired: 2 in, 2 out]
        n134 = property on="3 4" class="Bool (strict)"("Value"=w47) -> ()  [unwired: 2 in, 2 out]
        n135 = flat-sequence {
          tunnel: [w221] -> w86
          tunnel: [w220] -> w85
          tunnel: [w217] -> w76
          tunnel: [w219] -> w84
          tunnel: [w218] -> w83
          tunnel: ["Channel # 4"] -> w82
          tunnel: "VISA resource name 4" -> [w217]
          tunnel: w86 -> [w241]
          tunnel: w85 -> [w240]
          tunnel: [w239] -> w73
          tunnel: w84 -> [w239]
          tunnel: [w238] -> w74
          tunnel: w83 -> [w238]
          tunnel: [w237] -> w71
          tunnel: w82 -> [w237]
          frame #0 {
            w221 = 2730.0 ("Voltage Set (Volts)")
            w220 = 10.0 ("Voltage Ramp Up (V/s)")
            n136 = call <instrlib>:"Initialize.vi"("VISA resource name"=w217) -> ("error out"=w231:errorcluster, "VISA resource name out"=w227:refnum<visa-resource-name>)  [unwired: 9 in]
            n137 = call <instrlib>:"OpenBoard.vi"("error in (no error)"=w231, "Board Address"=0, "VISA resource name"=w227) -> ("error out"=w232:errorcluster, "BoardHandle"=w226:T1)  [unwired: 7 in]
            n138 = call <instrlib>:"Clear alarm signal.vi"("error in (no error)"=w232, "BoardHandle"=w226) -> ("error out"=w215:errorcluster, "BoardHandle out"=w214:T1)  [unwired: 8 in]
            n139 = call <instrlib>:"Configure IMON RANGE.vi"("error in (no error)"=w215, "IMon range (LOW)"="HIGH", "Channel (0)"="Channel # 4", "BoardHandle"=w214) -> ("error out"=w210:errorcluster, "BoardHandle out"=w211:T1)  [unwired: 6 in]
            n140 = call <instrlib>:"Configure MAXV.vi"("error in (no error)"=w210, "Voltage Max (0.0 V)"=3000.0 ("VMax (Volts)"), "Channel (0)"="Channel # 4", "BoardHandle"=w211) -> ("error out"=w233:errorcluster, "BoardHandle out"=w225:T1)  [unwired: 6 in]
            n141 = call <instrlib>:"Configure ISET.vi"("error in (no error)"=w233, "Current Limit (0.00 uA)"=20.0 ("Current Limit (uA)"), "Channel (0)"="Channel # 4", "BoardHandle"=w225) -> ("error out"=w234:errorcluster, "BoardHandle out"=w224:T1)  [unwired: 6 in]
            n142 = call <instrlib>:"Configure VSET.vi"("error in (no error)"=w234, "Voltage Level (0.0 V)"=w221, "Channel (0)"="Channel # 4", "BoardHandle"=w224) -> ("error out"=w235:errorcluster, "BoardHandle out"=w223:T1)  [unwired: 6 in]
            n143 = call <instrlib>:"Configure RAMP UP.vi"("error in (no error)"=w235, "Voltage ramp up (0 V/s)"=w220, "Channel (0)"="Channel # 4", "BoardHandle"=w223) -> ("error out"=w236:errorcluster, "BoardHandle out"=w222:T1)  [unwired: 6 in]
            n144 = call <instrlib>:"Channel Power Enable.vi"("error in (no error)"=w236, "Enable (OFF)"=TRUE ("Boolean"), "Channel (0)"="Channel # 4", "BoardHandle"=w222) -> ("error out"=w218:errorcluster, "BoardHandle out"=w219:T1)  [unwired: 6 in]
          }
          frame #1 {
            n145 = Divide(x=w241, y=w240) -> (x/y=w244:dbl)
            n146 = Add(x=w244, y=10.0) -> (x+y=w245:dbl)
            n147 = Multiply(x=w245, y=1000.0) -> (x*y=w246:dbl)
            n148 = Wait (ms)(milliseconds to wait=w246) -> ()  [unwired: 1 out]
          }
        }
        n149 = property on="Test is Running 4" class="Bool (strict)"("Value"=TRUE) -> ()  [unwired: 2 in, 2 out]
        n150 = call <instrlib>:"Configure IMON RANGE.vi"("error in (no error)"=w74, "IMon range (LOW)"="LOW", "Channel (0)"=w71, "BoardHandle"=w73) -> ("error out"=w69:errorcluster, "BoardHandle out"=w70:T1)  [unwired: 6 in]
        n151 = for {
          N: "N 4" -> [w255]
          tunnel: w69 -> [w262]
          tunnel: w71 -> [w263]
          tunnel: [w265] -> w80
          tunnel: [w264] -> w79
          tunnel: [w256] -> w48 mode=indexing
          tunnel: [w263] -> w77
          tunnel: w70 -> [w259]
          tunnel: [w262] -> _ mode=indexing
          tunnel: ["dt (s) 4"] -> w46
          i -> [w252]
          stop <- w250 stop-if-true
          n152 = call <instrlib>:"Channel Status.vi"("error in (no error)"=w262, "BoardHandle"=w259) -> ("error out"=w271:errorcluster, "Channel Status Array"=w275:T2, "BoardHandle out"=w270:T1)  [unwired: 7 in]
          n153 = Index Array(array=w275, index=w263) -> (element=w274:T3)
          n154 = call <instrlib>:"Read out VMON.vi"("error in (no error)"=w271, "BoardHandle"=w270) -> ("error out"=w267:errorcluster, "VMon values (V)"=w269:dbl[], "BoardHandle out"=w268:T1)  [unwired: 7 in]
          n155 = Unbundle By Name(w274) -> ("OVV"=→"OVV? 8":bool, "OVC"=→"OVC? 8":bool)
          n156 = Index Array(array=w269, index=w263) -> (element=w249:dbl)
          "Actual Voltage Level (V) 8" <- w249
          n157 = Increment(x=w252) -> (x+1=w251:i32)
          n158 = call <instrlib>:"Read out IMON.vi"("error in (no error)"=w267, "BoardHandle"=w268) -> ("error out"=w264:errorcluster, "IMon values (uA)"=w266:dbl[], "BoardHandle out"=w265:T1)  [unwired: 6 in, 1 out]
          n159 = Less?(x=w249, y=2000.0) -> (x < y?=w250:bool)
          "Power Supply Trip 4" <- w250
          n160 = Index Array(array=w266, index=w263) -> (element=w258:dbl)
          n161 = Subtract(x=w255, y=w251) -> (x-y=w254:i32)
          n162 = Multiply(x=w258, y=1000.0) -> (x*y=w256:dbl)
          "Actual Current Limit (nA) 4" <- w256
          n163 = Multiply(x=w254, y="dt (s) 4") -> (x*y=→"Time Left (s) 4":i32)
          n164 = Multiply(x="dt (s) 4", y=1000) -> (x*y=w261:i32)
          n165 = Wait (ms)(milliseconds to wait=w261) -> ()  [unwired: 1 out]
        }
        n166 = Format Into String(w46) -> (resulting string=w38:string)  [unwired: 3 in, 1 out]
        n167 = Array Size(array=w48) -> (size(s)=w68:i32)
        n168 = Decrement(x=w68) -> (x-1=w67:i32)
        n169 = Index Array(array=w48, index=w67) -> (element=w66:dbl)
        n170 = Greater?(x=8.0, y=w66) -> (0:w65:bool)
        n171 = Get Date/Time In Seconds() -> (seconds since 1Jan1904=w51:timestamp)
        n172 = Not(x=w65) -> (.not. x?=→"Manual Measurments \nNeeded 4":bool)
        n173 = String To Path(string="C:\\Users\\Swager\\Dropbox\\sMDT\\DarkCurrent") -> (path=w50:path)
        n174 = Format Date/Time String(time format string (%c)="data_%d_%m_%Y_%H_%M_%S.csv", seconds (now)=w51) -> (date/time string=w52:string)  [unwired: 1 in]
        n175 = Concatenate Strings(w38, "\r") -> (w39:string)
        n176 = Build Path(base path=w50, name or relative path=w52) -> (appended path=w41:path)
        n177 = flat-sequence {
          tunnel: w41 -> [w93]
          tunnel: [w93] -> w45
          tunnel: [w94] -> w43
          tunnel: w48 -> [w94]
          tunnel: w39 -> [w90]
          tunnel: w45 -> [w100]
          tunnel: [w100] -> w44
          tunnel: w43 -> [w99]
          tunnel: [w99] -> w42
          tunnel: w41 -> [w98]
          tunnel: "Barcodes 4" -> [w97]
          tunnel: w44 -> [w103]
          tunnel: w42 -> [w102]
          frame #0 {
            n178 = Open/Create/Replace File(file path (use dialog)=w93, operation (0:open)=2) -> (refnum out=w91:refnum<file>, error out=w92:errorcluster)  [unwired: 4 in, 1 out]
            n179 = Write to Text File(file (use dialog)=w91, text=w90, error in=w92) -> (refnum out=w88:refnum<file>, error out=w89:errorcluster)  [unwired: 1 in, 1 out]
            n180 = Close File(refnum=w88, error in=w89) -> ()  [unwired: 2 out]
          }
          frame #1 {
            n181 = call-poly <vilib>:"Write Delimited Spreadsheet.vi"("file path (dialog if empty)"=w98, "1D data"=w97, "append to file? (new file:F)"=TRUE, "delimiter (\\t)"=",") -> ()  [unwired: 10 in, 2 out]
          }
          frame #2 {
            n182 = call-poly <vilib>:"Write Delimited Spreadsheet.vi"("file path (dialog if empty)"=w103, "1D data"=w102, "append to file? (new file:F)"=TRUE, "transpose? (no:F)"=TRUE, "delimiter (\\t)"=",") -> ()  [unwired: 9 in, 2 out]
          }
        }
        n183 = case shown="False" w65 {
          tunnel: w80 -> [w132 w205]
          tunnel: w79 -> [w133 w204]
          tunnel: FALSE -> [_ _]
          tunnel: w77 -> [w131 w203]
          tunnel: w76 -> [w127 w206]
          tunnel: w48 -> [_ _]
          tunnel: "Barcodes 4" -> [w123 _]
          tunnel: [w113 w209] -> w61
          tunnel: [w112 w209] -> w60
          tunnel: [w111 w209] -> w59
          tunnel: [w110 w209] -> w58
          tunnel: [w109 w209] -> w57
          tunnel: [w108 w209] -> w56
          tunnel: [w107 w209] -> w55
          tunnel: [w106 w209] -> w54
          frame False {
            n184 = while {
              shift-right: [w139] -> w124
              shift-left: w131 -> [w149]
              shift-right: [w141] -> w126
              shift-left: w132 -> [w146]
              shift-right: [w140] -> w125
              shift-left: w133 -> [w144]
              tunnel: w123 -> [w137]
              tunnel: [w134] -> w122 mode=indexing
              i -> [w152]
              stop <- w153 stop-if-true
              n185 = flat-sequence {
                tunnel: w152 -> [w160]
                tunnel: [w159] -> w151
                tunnel: w149 -> [w158]
                tunnel: [w158] -> w148
                tunnel: [w157] -> w147
                tunnel: w146 -> [w157]
                tunnel: [w156] -> w145
                tunnel: w144 -> [w156]
                tunnel: w137 -> [w155]
                tunnel: w151 -> [w170]
                tunnel: [w170] -> w150
                tunnel: w148 -> [w165]
                tunnel: w147 -> [w168]
                tunnel: w145 -> [w169]
                tunnel: [w167] -> w143
                tunnel: [w166] -> w142
                tunnel: [w165] -> w139
                tunnel: [w164] -> w138
                tunnel: [w163] -> w136
                tunnel: w150 -> [w188]
                tunnel: w143 -> [w186]
                tunnel: w142 -> [w185]
                tunnel: [w186] -> w141
                tunnel: [w185] -> w140
                tunnel: w138 -> [w184]
                frame #0 {
                  n186 = while {
                    stop <- "Measure Next Tube 4" stop-if-true
                    n187 = Wait (ms)(milliseconds to wait=100) -> ()  [unwired: 1 out]
                  }
                  n188 = Index Array(array=w155, index=w160) -> (element=w159:string)
                  "Next Measurment 4" <- w159
                }
                frame #1 {
                  n189 = call <instrlib>:"Channel Status.vi"("error in (no error)"=w169, "BoardHandle"=w168) -> ("error out"=w176:errorcluster, "Channel Status Array"=w172:T2, "BoardHandle out"=w177:T1)  [unwired: 7 in]
                  n190 = Index Array(array=w172, index=w165) -> (element=w173:T3)
                  n191 = call <instrlib>:"Read out VMON.vi"("error in (no error)"=w176, "BoardHandle"=w177) -> ("error out"=w180:errorcluster, "VMon values (V)"=w178:dbl[], "BoardHandle out"=w179:T1)  [unwired: 7 in]
                  n192 = Unbundle By Name(w173) -> ("OVV"=→"OVV? 7":bool, "OVC"=→"OVC? 7":bool)
                  n193 = Index Array(array=w178, index=w165) -> (element=→"Actual Voltage Level (V) 7":dbl)
                  n194 = call <instrlib>:"Read out IMON.vi"("error in (no error)"=w180, "BoardHandle"=w179) -> ("error out"=w166:errorcluster, "IMon values (uA)"=w183:dbl[], "BoardHandle out"=w167:T1)  [unwired: 6 in, 1 out]
                  n195 = Index Array(array=w183, index=w165) -> (element=w181:dbl)
                  n196 = Multiply(x=w181, y=1000.0) -> (x*y=w163:dbl)
                  "Recorded Current\nfor Previous Tube 4" <- w163
                  n197 = Format Into String(w163) -> (resulting string=w164:string)  [unwired: 3 in, 1 out]
                }
                frame #2 {
                  n198 = Get Date/Time In Seconds() -> (seconds since 1Jan1904=w200:timestamp)
                  n199 = String To Path(string="C:\\Users\\Swager\\Dropbox\\sMDT\\DarkCurrent") -> (path=w199:path)
                  n200 = Format Date/Time String(time format string (%c)="data_%d_%m_%Y_%H_%M_%S.csv", seconds (now)=w200) -> (date/time string=w201:string)  [unwired: 1 in]
                  n201 = Build Path(base path=w199, name or relative path=w201) -> (appended path=w197:path)
                  n202 = Open/Create/Replace File(file path (use dialog)=w197, operation (0:open)=5) -> (refnum out=w196:refnum<file>, error out=w195:errorcluster)  [unwired: 4 in, 1 out]
                  n203 = Concatenate Strings(w188, "\r\n", w184, ",") -> (w190:string)
                  n204 = Write to Text File(file (use dialog)=w196, text=w190, error in=w195) -> (refnum out=w194:refnum<file>, error out=w193:errorcluster)  [unwired: 1 in, 1 out]
                  n205 = Close File(refnum=w194, error in=w193) -> (error out=w192:errorcluster)  [unwired: 1 out]
                  n206 = call <vilib>:"Simple Error Handler.vi"("error in (no error)"=w192) -> ()  [unwired: 4 in, 5 out]
                }
              }
              n207 = Greater?(x=w152, y=6) -> (0:w153:bool)
              n208 = Less?(x=w136, y=2.0) -> (x < y?=w134:bool)
            }
            n209 = Index Array(array=w122, index=1) -> (element=w112:bool)
            n210 = Index Array(array=w122, index=3) -> (element=w110:bool)
            n211 = Index Array(array=w122, index=4) -> (element=w109:bool)
            n212 = Index Array(array=w122, index=5) -> (element=w108:bool)
            n213 = Index Array(array=w122, index=6) -> (element=w107:bool)
            n214 = Index Array(array=w122, index=7) -> (element=w106:bool)
            n215 = call <instrlib>:"Channel Power Enable.vi"("error in (no error)"=w125, "Enable (OFF)"=FALSE, "Channel (0)"=w124, "BoardHandle"=w126) -> ("error out"=w129:errorcluster)  [unwired: 6 in, 1 out]
            n216 = Index Array(array=w122, index=0) -> (element=w113:bool)
            n217 = Index Array(array=w122, index=2) -> (element=w111:bool)
            n218 = call <instrlib>:"Close.vi"("error in (no error)"=w129, "VISA resource name"=w127) -> ("error out"=w128:errorcluster)  [unwired: 9 in]
            n219 = call <vilib>:"Simple Error Handler.vi"("error in (no error)"=w128) -> ()  [unwired: 4 in, 5 out]
          }
          frame True {
            w209 = TRUE
            n220 = call <instrlib>:"Channel Power Enable.vi"("error in (no error)"=w204, "Channel (0)"=w203, "BoardHandle"=w205) -> ("error out"=w208:errorcluster)  [unwired: 7 in, 1 out]
            n221 = call <instrlib>:"Close.vi"("error in (no error)"=w208, "VISA resource name"=w206) -> ("error out"=w207:errorcluster)  [unwired: 9 in]
            n222 = call <vilib>:"Simple Error Handler.vi"("error in (no error)"=w207) -> ()  [unwired: 4 in, 5 out]
          }
        }
      }
    }
    n223 = flat-sequence {
      tunnel: [w541] -> w24
      tunnel: [w540] -> w23
      tunnel: [w539] -> w22
      tunnel: [w538] -> w21
      tunnel: [w537] -> w20
      tunnel: [w536] -> w19
      tunnel: [w535] -> w18
      tunnel: [w534] -> w17
      frame #0 {
        w518 = FALSE
        n224 = while {
          stop <- "Begin Test 2" stop-if-true
          n225 = Wait (ms)(milliseconds to wait=100) -> ()  [unwired: 1 out]
        }
        n226 = property on="Manual Measurments \nNeeded 2" class="Bool (strict)"("Value"=w518) -> ()  [unwired: 2 in, 2 out]
        n227 = property on="Test is Running 2" class="Bool (strict)"("Value"=w518) -> ()  [unwired: 2 in, 2 out]
      }
      frame #1 {
        w532 = FALSE
        n228 = property on="Power Supply Trip 2" class="Bool (strict)"("Value"=w532) -> ()  [unwired: 2 in, 2 out]
        n229 = property on="1 2" class="Bool (strict)"("Value"=w532) -> ()  [unwired: 2 in, 2 out]
        n230 = property on="2 2" class="Bool (strict)"("Value"=w532) -> ()  [unwired: 2 in, 2 out]
        n231 = property on="4 2" class="Bool (strict)"("Value"=w532) -> ()  [unwired: 2 in, 2 out]
        n232 = property on="7 2" class="Bool (strict)"("Value"=w532) -> ()  [unwired: 2 in, 2 out]
        n233 = property on="5 2" class="Bool (strict)"("Value"=w532) -> ()  [unwired: 2 in, 2 out]
        n234 = property on="6 2" class="Bool (strict)"("Value"=w532) -> ()  [unwired: 2 in, 2 out]
        n235 = property on="8 2" class="Bool (strict)"("Value"=w532) -> ()  [unwired: 2 in, 2 out]
        n236 = property on="3 2" class="Bool (strict)"("Value"=w532) -> ()  [unwired: 2 in, 2 out]
        n237 = property on="Test is Running 2" class="Bool (strict)"("Value"=TRUE) -> ()  [unwired: 2 in, 2 out]
        n238 = call "Channel 1-1 First Half (SubVI).vi"("VISA Refnum in"="VISA resource name 2", "Channel # in"="Channel # 2", "dt (s) in"="dt (s) 2", "Barcodes in"="Barcodes 2", "N in"="N 2") -> ("Actual Voltage Level (V) 4"=→"Actual Voltage Level (V) 4":dbl, "OVV? 4"=→"OVV? 4":bool, "Power Supply Trip 2"=→"Power Supply Trip 2":bool, "OVC? 4"=→"OVC? 4":bool, "Boolean 2"=w547:bool, "Actual Current Limit (nA) 2"=→"Actual Current Limit (nA) 2":dbl, "BoardHandle out 2"=w549:T1, "VISA Refnum out"=w545:refnum<visa-resource-name>, "Time Left (s) 2"=→"Time Left (s) 2":dbl, "Manual Measurments \nNeeded 2"=→"Manual Measurments \nNeeded 2":bool, "Barcodes 3"=w531:string[], "Boolean"=w543:bool, "Channel # 4"=w546:i32, "Array"=w533:dbl[], "error out"=w548:errorcluster)  [unwired: 8 in]
        n239 = case shown="False" w543 {
          tunnel: w549 -> [w577 w650]
          tunnel: w548 -> [w578 w649]
          tunnel: w547 -> [_ _]
          tunnel: w546 -> [w576 w648]
          tunnel: w545 -> [w572 w651]
          tunnel: w533 -> [_ _]
          tunnel: w531 -> [w568 _]
          tunnel: [w558 w654] -> w541
          tunnel: [w557 w654] -> w540
          tunnel: [w556 w654] -> w539
          tunnel: [w555 w654] -> w538
          tunnel: [w554 w654] -> w537
          tunnel: [w553 w654] -> w536
          tunnel: [w552 w654] -> w535
          tunnel: [w551 w654] -> w534
          frame False {
            n240 = while {
              shift-right: [w584] -> w569
              shift-left: w576 -> [w594]
              shift-right: [w586] -> w571
              shift-left: w577 -> [w591]
              shift-right: [w585] -> w570
              shift-left: w578 -> [w589]
              tunnel: w568 -> [w582]
              tunnel: [w579] -> w567 mode=indexing
              i -> [w597]
              stop <- w598 stop-if-true
              n241 = flat-sequence {
                tunnel: w597 -> [w605]
                tunnel: [w604] -> w596
                tunnel: w594 -> [w603]
                tunnel: [w603] -> w593
                tunnel: [w602] -> w592
                tunnel: w591 -> [w602]
                tunnel: [w601] -> w590
                tunnel: w589 -> [w601]
                tunnel: w582 -> [w600]
                tunnel: w596 -> [w615]
                tunnel: [w615] -> w595
                tunnel: w593 -> [w610]
                tunnel: w592 -> [w613]
                tunnel: w590 -> [w614]
                tunnel: [w612] -> w588
                tunnel: [w611] -> w587
                tunnel: [w610] -> w584
                tunnel: [w609] -> w583
                tunnel: [w608] -> w581
                tunnel: w595 -> [w633]
                tunnel: w588 -> [w631]
                tunnel: w587 -> [w630]
                tunnel: [w631] -> w586
                tunnel: [w630] -> w585
                tunnel: w583 -> [w629]
                frame #0 {
                  n242 = while {
                    stop <- "Measure Next Tube 2" stop-if-true
                    n243 = Wait (ms)(milliseconds to wait=100) -> ()  [unwired: 1 out]
                  }
                  n244 = Index Array(array=w600, index=w605) -> (element=w604:string)
                  "Next Measurment 2" <- w604
                }
                frame #1 {
                  n245 = call <instrlib>:"Channel Status.vi"("error in (no error)"=w614, "BoardHandle"=w613) -> ("error out"=w621:errorcluster, "Channel Status Array"=w617:T2, "BoardHandle out"=w622:T1)  [unwired: 7 in]
                  n246 = Index Array(array=w617, index=w610) -> (element=w618:T3)
                  n247 = call <instrlib>:"Read out VMON.vi"("error in (no error)"=w621, "BoardHandle"=w622) -> ("error out"=w625:errorcluster, "VMon values (V)"=w623:dbl[], "BoardHandle out"=w624:T1)  [unwired: 7 in]
                  n248 = Unbundle By Name(w618) -> ("OVV"=→"OVV? 3":bool, "OVC"=→"OVC? 3":bool)
                  n249 = Index Array(array=w623, index=w610) -> (element=→"Actual Voltage Level (V) 3":dbl)
                  n250 = call <instrlib>:"Read out IMON.vi"("error in (no error)"=w625, "BoardHandle"=w624) -> ("error out"=w611:errorcluster, "IMon values (uA)"=w628:dbl[], "BoardHandle out"=w612:T1)  [unwired: 6 in, 1 out]
                  n251 = Index Array(array=w628, index=w610) -> (element=w626:dbl)
                  n252 = Multiply(x=w626, y=1000.0) -> (x*y=w608:dbl)
                  "Recorded Current\nfor Previous Tube 2" <- w608
                  n253 = Format Into String(w608) -> (resulting string=w609:string)  [unwired: 3 in, 1 out]
                }
                frame #2 {
                  n254 = Get Date/Time In Seconds() -> (seconds since 1Jan1904=w645:timestamp)
                  n255 = String To Path(string="C:\\Users\\Swager\\Dropbox\\sMDT\\DarkCurrent") -> (path=w644:path)
                  n256 = Format Date/Time String(time format string (%c)="data_%d_%m_%Y_%H_%M_%S.csv", seconds (now)=w645) -> (date/time string=w646:string)  [unwired: 1 in]
                  n257 = Build Path(base path=w644, name or relative path=w646) -> (appended path=w642:path)
                  n258 = Open/Create/Replace File(file path (use dialog)=w642, operation (0:open)=5) -> (refnum out=w641:refnum<file>, error out=w640:errorcluster)  [unwired: 4 in, 1 out]
                  n259 = Concatenate Strings(w633, "\r\n", w629, ",") -> (w635:string)
                  n260 = Write to Text File(file (use dialog)=w641, text=w635, error in=w640) -> (refnum out=w639:refnum<file>, error out=w638:errorcluster)  [unwired: 1 in, 1 out]
                  n261 = Close File(refnum=w639, error in=w638) -> (error out=w637:errorcluster)  [unwired: 1 out]
                  n262 = call <vilib>:"Simple Error Handler.vi"("error in (no error)"=w637) -> ()  [unwired: 4 in, 5 out]
                }
              }
              n263 = Greater?(x=w597, y=6) -> (0:w598:bool)
              n264 = Less?(x=w581, y=2.0) -> (x < y?=w579:bool)
            }
            n265 = Index Array(array=w567, index=1) -> (element=w557:bool)
            n266 = Index Array(array=w567, index=3) -> (element=w555:bool)
            n267 = Index Array(array=w567, index=4) -> (element=w554:bool)
            n268 = Index Array(array=w567, index=5) -> (element=w553:bool)
            n269 = Index Array(array=w567, index=6) -> (element=w552:bool)
            n270 = Index Array(array=w567, index=7) -> (element=w551:bool)
            n271 = call <instrlib>:"Channel Power Enable.vi"("error in (no error)"=w570, "Enable (OFF)"=FALSE, "Channel (0)"=w569, "BoardHandle"=w571) -> ("error out"=w574:errorcluster)  [unwired: 6 in, 1 out]
            n272 = Index Array(array=w567, index=0) -> (element=w558:bool)
            n273 = Index Array(array=w567, index=2) -> (element=w556:bool)
            n274 = call <instrlib>:"Close.vi"("error in (no error)"=w574, "VISA resource name"=w572) -> ("error out"=w573:errorcluster)  [unwired: 9 in]
            n275 = call <vilib>:"Simple Error Handler.vi"("error in (no error)"=w573) -> ()  [unwired: 4 in, 5 out]
          }
          frame True {
            w654 = TRUE
            n276 = call <instrlib>:"Channel Power Enable.vi"("error in (no error)"=w649, "Channel (0)"=w648, "BoardHandle"=w650) -> ("error out"=w653:errorcluster)  [unwired: 7 in, 1 out]
            n277 = call <instrlib>:"Close.vi"("error in (no error)"=w653, "VISA resource name"=w651) -> ("error out"=w652:errorcluster)  [unwired: 9 in]
            n278 = call <vilib>:"Simple Error Handler.vi"("error in (no error)"=w652) -> ()  [unwired: 4 in, 5 out]
          }
        }
      }
    }
    "1" <- w32
    "2" <- w31
    "3" <- w30
    "4" <- w29
    "5" <- w28
    "8" <- w25
    "6" <- w27
    "7" <- w26
    "1 2" <- w24
    "2 2" <- w23
    "3 2" <- w22
    "4 2" <- w21
    "5 2" <- w20
    "8 2" <- w17
    "6 2" <- w19
    "7 2" <- w18
    "1 3" <- w16
    "2 3" <- w15
    "3 3" <- w14
    "4 3" <- w13
    "5 3" <- w12
    "8 3" <- w9
    "6 3" <- w11
    "7 3" <- w10
    "1 4" <- w8
    "2 4" <- w7
    "3 4" <- w6
    "4 4" <- w5
    "5 4" <- w4
    "8 4" <- w1
    "6 4" <- w3
    "7 4" <- w2
  }
